vi "Read Attributes.vi"(11 "CapturedImage Msg":refnum<class "CapturedImage Msg.lvclass">) -> (2 "Payload":cluster{"JSON":string})   [LabVIEW 2021, in "Vision.lvlib" / "CapturedImage Msg.lvclass"]
uses:
  CapturedImage Msg.lvclass
  CapturedImage Msg.lvclass/CapturedImage Msg.ctl
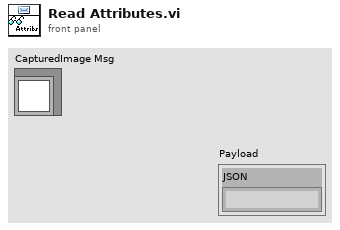
[diagram p1: front panel]
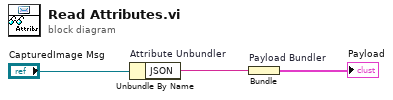
[diagram p0: block diagram]
diagram:
  n1 = Unbundle By Name "Attribute Unbundler"("CapturedImage Msg") -> ("JSON"=w1:string)
  n2 = Bundle "Payload Bundler"("JSON"=w1) -> (→"Payload":cluster{"JSON":string})  [unwired: 1 in]
